vi "Connect.vi"(8 "error in (no error)":errorcluster, 11 "TCP_Server in":refnum<class "TCP_Server.lvclass">) -> (0 "error out":errorcluster, 3 "TCP_Server out":refnum<class "TCP_Server.lvclass">)   [LabVIEW 2018, in "TCP_Server.lvlib" / "TCP_Server.lvclass"]
uses:
  TCP_Server.lvclass
  C:/Repos/AF_TCP_Example/TCP_Client/TCP_Client/TCP_Client.lvclass
  TCP_Client/TCP_Client/TCP_Client.lvclass/TCP_Client.ctl
  TCP_Client/TCP_Client/Accessor/Read port.vi
  TCP_Client/TCP_Client/Accessor/Read timeout ms.vi
  TCP_Client/TCP_Client/Accessor/Write connection ID.vi
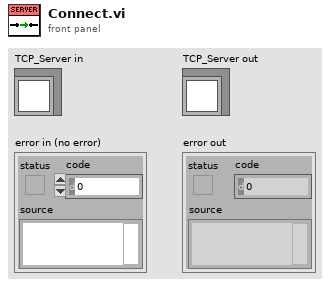
[diagram p1: front panel]
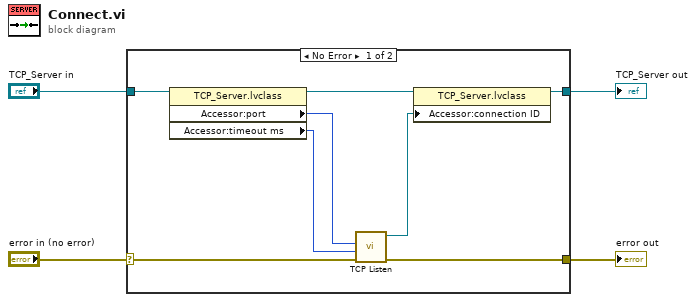
[diagram p0: block diagram]
diagram:
  n1 = case shown="No Error" "error in (no error)" {
    selector: "error in (no error)" -> [w12 w13]
    tunnel: [w11 w13] -> w3
    tunnel: "TCP_Server in" -> [w10 w14]
    tunnel: [w6 w14] -> w1
    frame No Error {
      n2 = property class="TCP_Server.lvclass"(reference=w10) -> (reference out=w9:refnum<class "TCP_Server.lvclass">, "Accessor:port"=w8:u16, "Accessor:timeout ms"=w7:i32)  [unwired: 1 in, 1 out]
      n3 = call <vilib>:"TCP Listen.vi"("error in (no error)"=w12, "timeout ms (wait forever: -1)"=w7, "port"=w8) -> ("error out"=w11:errorcluster, "connection ID"=w5:refnum<k5>)  [unwired: 4 in, 3 out]
      n4 = property class="TCP_Server.lvclass"(reference=w9, "Accessor:connection ID"=w5) -> (reference out=w6:refnum<class "TCP_Server.lvclass">)  [unwired: 1 in, 1 out]
    }
    frame Error {
    }
  }
  "error out" <- w3
  "TCP_Server out" <- w1
